vi "queueAcq.vi"(6 "table":T1(ring), 8 "error in (no error)":errorcluster, 9 "Window Number (0...15)":i32, 10 "period_type":string="none", 11 "Acquisition in":refnum<class "Acquisition.lvclass">) -> (0 "error out":errorcluster, 2 "current time":timestamp, 3 "Acquisition out":refnum<class "Acquisition.lvclass">)   [LabVIEW 2014, in "Acquisition.lvclass"]
uses:
  Acquisition.lvclass
  Acquisition.lvclass/Acquisition.ctl
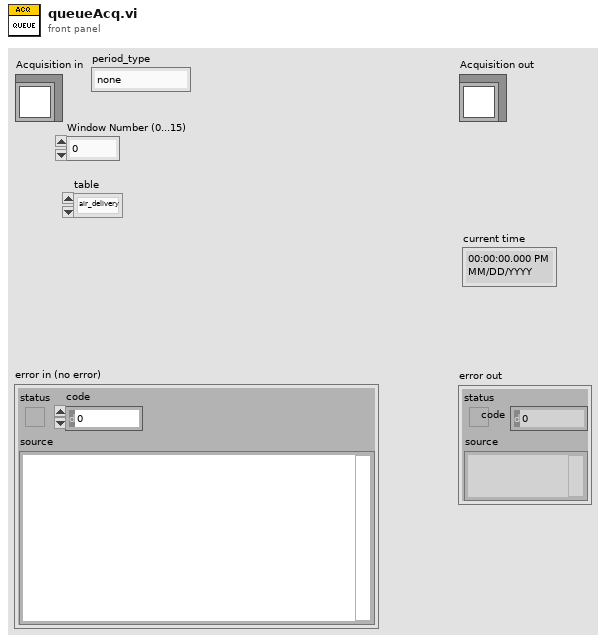
[diagram p1: front panel]
types:
  T1 = enum16{"air_delivery", "beh_session", "stim_periods", "licks", "liquid_delivery", ""}
  T2 = cluster{"table":enum16{"air_delivery", "beh_session", "stim_periods", "licks", "liquid_delivery"}, "timestamp":dbl, "Window Number (0...15)":i32, "period_type":string}
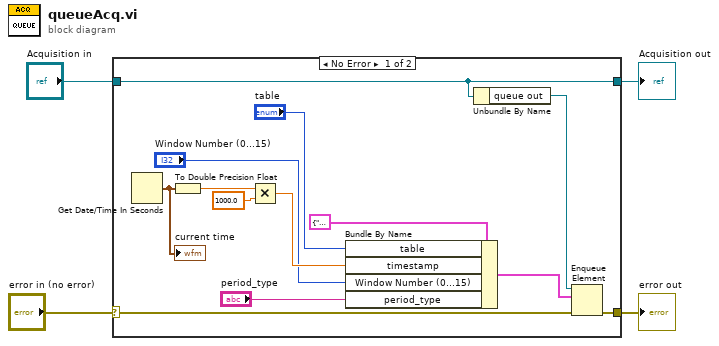
[diagram p0: block diagram]
diagram:
  n1 = case shown="No Error" "error in (no error)" {
    selector: "error in (no error)" -> [w14 w19]
    tunnel: [w13 w19] -> w3
    tunnel: [w11 w18] -> w1
    tunnel: "Acquisition in" -> [w11 w18]
    frame No Error {
      n2 = Get Date/Time In Seconds() -> (seconds since 1Jan1904=w15:timestamp)
      "current time" <- w15
      n3 = To Double Precision Float(number=w15) -> (double precision float=w16:dbl)
      n4 = Multiply(x=w16, y=1000.0) -> (x*y=w12:dbl)
      n5 = Bundle By Name(cluster=T2 {"table"=enum."air_delivery", "timestamp"=0.0, "Window Number (0...15)"=0, "period_type"=""} ("element"), "table"="table", "timestamp"=w12, "Window Number (0...15)"="Window Number (0...15)", "period_type"="period_type") -> (w5:T2)
      n6 = Unbundle By Name(w11) -> ("queue out"=w10:refnum<queue>)
      n7 = Enqueue Element(queue=w10, element=w5, error in (no error)=w14) -> (error out=w13:errorcluster)  [unwired: 1 in, 2 out]
    }
    frame Error {
    }
  }
  "error out" <- w3
  "Acquisition out" <- w1
